vi "总磷氨氮插入数据.vi"(0 "table":string, 1 "关键参数":T1, 5 "data":T2={"时间标识"=timestamp(0 s since 1904-01-01), "测量模式"=enum."水样测试", "数据标记表"="N", "监测值"=0.0, "单位"=0, "数据标识"="", "因子编码"=0, "标样参考值"=0.0, "F0"=0.0, "F1"=0.0, "F2"=0.0, "F3"=0.0, "F4"=0.0, "F5"=0.0, "F6"=0.0, "F7"=0.0, "X"=0.0, "温度"=0.0, "湿度"=0.0, "量程标识"="", "SN"="", "跨度值"=0.0, "X1"=0.0} {"单位" items=["μg/L", "mg/L", "ppm", "mg/m3", "cm", "ppb", "μg/m3", "%", "nmol/mol", "μmol/mol", "MPN/L", "MPN/100ml", "ng/m3", "NTU", "无量纲", "ms/cm", "μs/cm"]}, 11 "error in (no error)":errorcluster) -> (15 "error out":errorcluster)   [LabVIEW 2016, in "斯坦道总氮.lvlib"]
uses:
  <vilib>/Utility/error.llb/DialogType.ctl
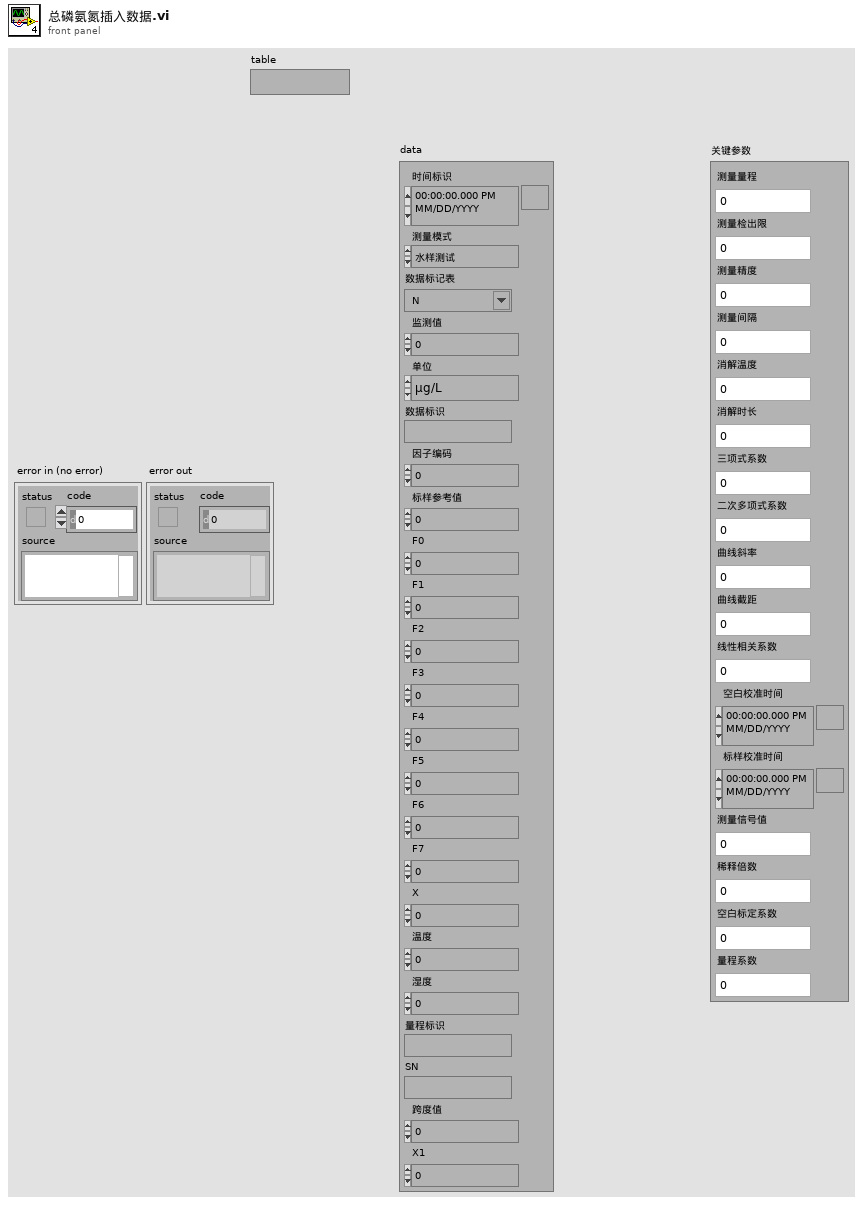
[diagram p1: front panel]
types:
  T1 = typedef "斯坦道总氮.lvlib/关键参数.ctl" = cluster{"测量量程":sgl, "测量检出限":sgl, "测量精度":sgl, "测量间隔":sgl, "消解温度":sgl, "消解时长":sgl, "三项式系数":sgl, "二次多项式系数":sgl, "曲线斜率":sgl, "曲线截距":sgl, "线性相关系数":sgl, "空白校准时间":timestamp, "标样校准时间":timestamp, "测量信号值":sgl, "稀释倍数":sgl, "空白标定系数":sgl, "量程系数":sgl}
  T2 = cluster{"时间标识":timestamp, "测量模式":enum16{"维护数据", "水样测试", "标样核查", "零点核查", "跨度核查", "空白测试", "平行样测试", "加标回收", "空白校准", "标样校准", "初始化（清洗）", "快捷测试"}, "数据标记表":string, "监测值":sgl, "单位":u16, "数据标识":string, "因子编码":u32, "标样参考值":sgl, "F0":sgl, "F1":sgl, "F2":sgl, "F3":sgl, "F4":sgl, "F5":sgl, "F6":sgl, "F7":sgl, "X":sgl, "温度":sgl, "湿度":sgl, "量程标识":string, "SN":string, "跨度值":sgl, "X1":sgl}
  T3 = typedef "DialogType.ctl" = u16
  T4 = typedef "营养盐字段定义.ctl" = cluster{"时间":timestamp, "测量模式":string, "数据类型":string, "检测值":sgl, "单位":string, "数据标识":string, "X":sgl, "量程标识":string, "SN":string, "标样参考值":sgl, "跨度值":sgl, "F0":sgl, "F1":sgl, "F2":sgl, "F3":sgl, "F4":sgl, "F5":sgl, "F6":sgl, "F7":sgl, "X1":sgl, "因子编码":string, "温度":sgl, "湿度":sgl, "测量量程":sgl, "测量检出限":sgl, "测量精度":sgl, "测量间隔":sgl, "消解温度":sgl, "消解时长":sgl, "三项式系数":sgl, "二次多项式系数":sgl, "曲线斜率":sgl, "曲线截距":sgl, "线性相关系数":sgl, "空白校准时间":timestamp, "标样校准时间":timestamp, "测量信号值":sgl, "稀释倍数":sgl, "空白标定系数":sgl, "量程系数":sgl, "LastTime":timestamp}
  T5 = typedef "数据库类型.ctl" = enum16{"Access", "SQLite"}
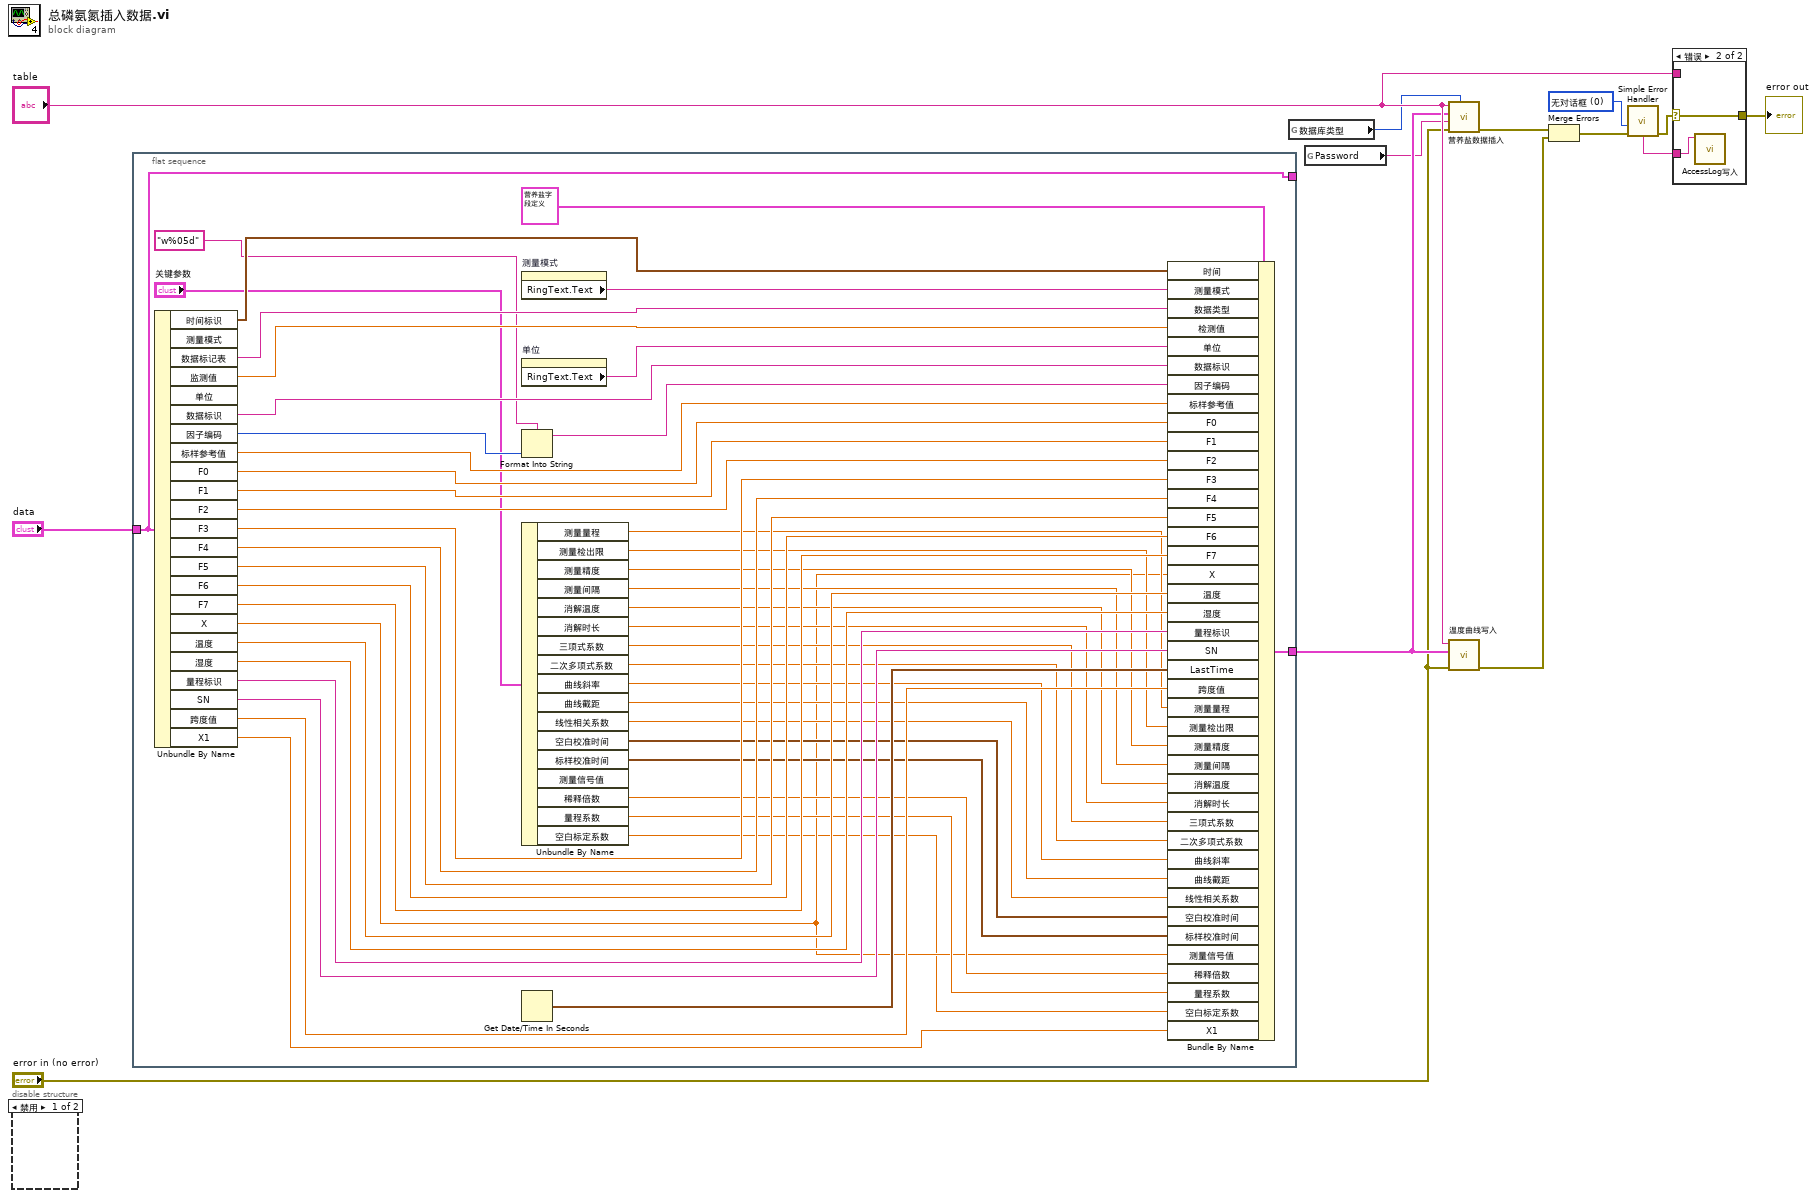
[diagram p0: block diagram]
diagram:
  w13 = T3 0 items=["无对话框", "确定信息", "继续或停止信息", "确定信息＋警告", "继续/停止+警告"] ("type of dialog (OK msg:1)")
  n1 = disable-structure shown="禁用" {
    frame Disabled {
    }
    frame Enabled {
    }
  }
  n2 = flat-sequence {
    tunnel: "data" -> [w39]
    tunnel: [w39] -> _
    tunnel: [w14] -> w6
    frame #0 {
      n3 = Unbundle By Name(w39) -> ("时间标识"=w59:timestamp, "数据标记表"=w57:string, "监测值"=w56:sgl, "数据标识"=w54:string, "因子编码"=w38:u32, "标样参考值"=w53:sgl, "F0"=w52:sgl, "F1"=w51:sgl, "F2"=w50:sgl, "F3"=w49:sgl, "F4"=w48:sgl, "F5"=w47:sgl, "F6"=w46:sgl, "F7"=w45:sgl, "X"=w18:sgl, "温度"=w44:sgl, "湿度"=w43:sgl, "量程标识"=w42:string, "SN"=w41:string, "跨度值"=w35:sgl, "X1"=w16:sgl)  [unwired: 2 out]
      n4 = property on="测量模式" class="Enum (严格)"() -> ("RingText.Text"=w58:string)  [unwired: 2 in, 2 out]
      n5 = property on="单位" class="Ring (严格)"() -> ("RingText.Text"=w55:string)  [unwired: 2 in, 2 out]
      n6 = Format Into String(format string="w%05d" ("格式字符串"), w38) -> (resulting string=w36:string)  [unwired: 2 in, 1 out]
      n7 = Unbundle By Name("关键参数") -> ("测量量程"=w33:sgl, "测量检出限"=w32:sgl, "测量精度"=w31:sgl, "测量间隔"=w30:sgl, "消解温度"=w29:sgl, "消解时长"=w28:sgl, "三项式系数"=w27:sgl, "二次多项式系数"=w26:sgl, "曲线斜率"=w25:sgl, "曲线截距"=w24:sgl, "线性相关系数"=w23:sgl, "空白校准时间"=w22:timestamp, "标样校准时间"=w21:timestamp, "稀释倍数"=w20:sgl, "量程系数"=w19:sgl, "空白标定系数"=w17:sgl)  [unwired: 1 out]
      n8 = Get Date/Time In Seconds() -> (seconds since 1Jan1904=w40:timestamp)
      n9 = Bundle By Name(cluster=T4 {"时间"=timestamp(0 s since 1904-01-01), "测量模式"="水样测试", "数据类型"="N", "检测值"=0.0, "单位"="mg/L", "数据标识"="N", "X"=0.0, "量程标识"="", "SN"="", "标样参考值"=0.0, "跨度值"=0.0, "F0"=0.0, "F1"=0.0, "F2"=0.0, "F3"=0.0, "F4"=0.0, "F5"=0.0, "F6"=0.0, "F7"=0.0, "X1"=0.0, "因子编码"="", "温度"=0.0, "湿度"=0.0, "测量量程"=0.0, "测量检出限"=0.0, "测量精度"=0.0, "测量间隔"=0.0, "消解温度"=0.0, "消解时长"=0.0, "三项式系数"=0.0, "二次多项式系数"=0.0, "曲线斜率"=0.0, "曲线截距"=0.0, "线性相关系数"=0.0, "空白校准时间"=timestamp(0 s since 1904-01-01), "标样校准时间"=timestamp(0 s since 1904-01-01), "测量信号值"=0.0, "稀释倍数"=0.0, "空白标定系数"=0.0, "量程系数"=0.0, "LastTime"=timestamp(0 s since 1904-01-01)} ("data"), "时间"=w59, "测量模式"=w58, "数据类型"=w57, "检测值"=w56, "单位"=w55, "数据标识"=w54, "因子编码"=w36, "标样参考值"=w53, "F0"=w52, "F1"=w51, "F2"=w50, "F3"=w49, "F4"=w48, "F5"=w47, "F6"=w46, "F7"=w45, "X"=w18, "温度"=w44, "湿度"=w43, "量程标识"=w42, "SN"=w41, "LastTime"=w40, "跨度值"=w35, "测量量程"=w33, "测量检出限"=w32, "测量精度"=w31, "测量间隔"=w30, "消解温度"=w29, "消解时长"=w28, "三项式系数"=w27, "二次多项式系数"=w26, "曲线斜率"=w25, "曲线截距"=w24, "线性相关系数"=w23, "空白校准时间"=w22, "标样校准时间"=w21, "测量信号值"=w18, "稀释倍数"=w20, "量程系数"=w19, "空白标定系数"=w17, "X1"=w16) -> (w14:T4)
    }
  }
  n10 = global read "总磷总氮断电保存全局变量.vi" "数据库类型"() -> (w2:T5)
  n11 = global read "总磷总氮断电保存全局变量.vi" "Password"() -> (w1:string)
  n12 = call "营养盐数据插入.vi"("Tabe Name"="table", "data"=w6, "Password"=w1, "错误输入（无错误）"="error in (no error)", "数据库类型"=w2) -> ("错误输出"=w8:errorcluster)  [unwired: 5 in]
  n13 = call "温度曲线写入.vi"("error in (no error)"="error in (no error)", "columns"=w6, "table"="table") -> ("错误输出"=w3:errorcluster)  [unwired: 8 in]
  n14 = Merge Errors(w8, w3) -> (w4:errorcluster)
  n15 = call <vilib>:"Simple Error Handler.vi"("type of dialog (OK msg:1)"=w13, "error in (no error)"=w4) -> ("error out"=w12:errorcluster, "message"=w11:string)  [unwired: 3 in, 3 out]
  n16 = case shown="错误" w12 {
    selector: w12 -> [_ w60]
    tunnel: w11 -> [_ w61]
    tunnel: [_ w60] -> w10
    tunnel: "table" -> [_ _]
    frame No Error {
    }
    frame Error {
      n17 = call "AccessLog写入.vi"("Log"=w61) -> ()  [unwired: 11 in]
    }
  }
  "error out" <- w10
